vi "Subtract Coinc Stats.vi"(8 "Statistics to remove":T1, 11 "Existing statistics":i32[][](array[numeric])) -> (3 "Output":i32[][](array[numeric]))   [LabVIEW 2016]
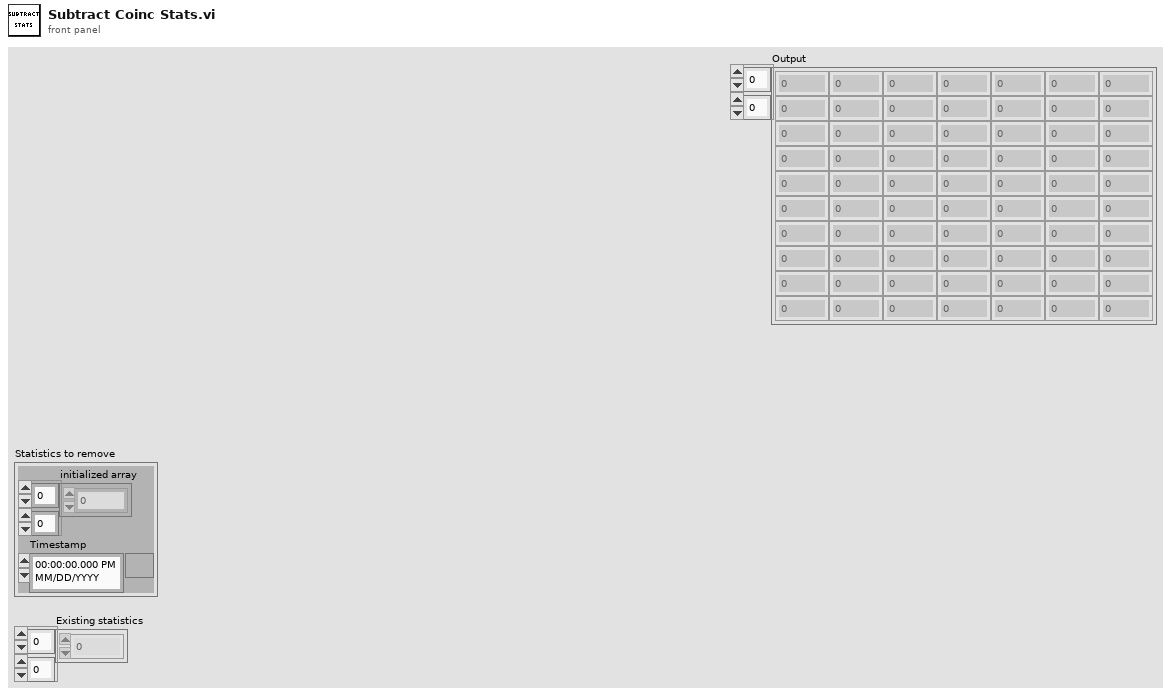
[diagram p1: front panel]
types:
  T1 = cluster{"initialized array":i16[][], "Timestamp":timestamp}
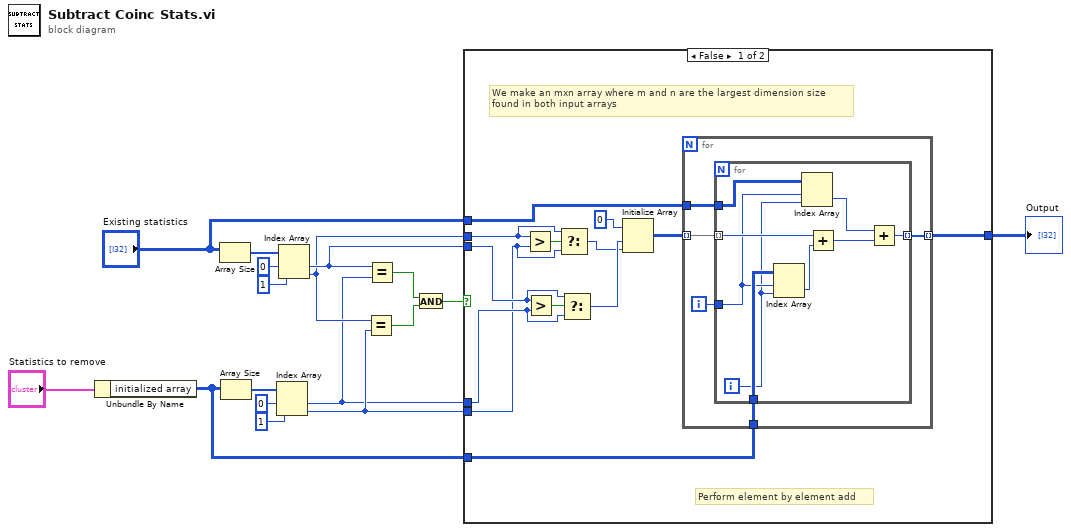
[diagram p0: block diagram]
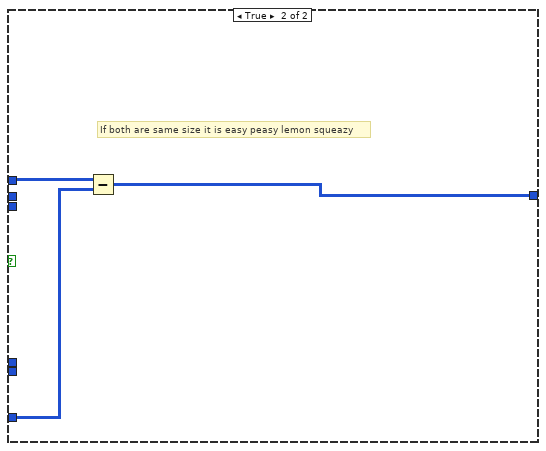
[diagram p2: hidden frame]
diagram:
  n1 = Unbundle By Name("Statistics to remove") -> ("initialized array"=w2:i16[][])
  n2 = Array Size(array="Existing statistics") -> (size(s)=w16:i32[])
  n3 = Array Size(array=w2) -> (size(s)=w11:i32[])
  n4 = Index Array(array=w11, index #1=0 ("index"), index #2=1 ("index")) -> (element #1=w4:i32, element #2=w5:i32)
  n5 = Index Array(array=w16, index #1=0 ("index"), index #2=1 ("index")) -> (element #1=w7:i32, element #2=w6:i32)
  n6 = Equal?(x=w6, y=w5) -> (x = y?=w9:bool)
  n7 = Equal?(x=w7, y=w4) -> (x = y?=w10:bool)
  n8 = And(x=w10, y=w9) -> (x .and. y?=w8:bool)
  n9 = case shown="False" w8 {
    tunnel: "Existing statistics" -> [w18 w47]
    tunnel: w2 -> [w20 w46]
    tunnel: [w19 w45] -> w1
    tunnel: w7 -> [w29 _]
    tunnel: w6 -> [w26 _]
    tunnel: w5 -> [w25 _]
    tunnel: w4 -> [w28 _]
    frame False {
      # "Perform element by element add"
      # "We make an mxn array where m and n are the largest dimension size\nfound in both input arrays"
      n10 = Greater?(x=w26, y=w25) -> (0:w27:bool)
      n11 = Greater?(x=w29, y=w28) -> (0:w30:bool)
      n12 = Select(t=w26, s=w27, f=w25) -> (s? t:f=w22:i32)
      n13 = Select(t=w29, s=w30, f=w28) -> (s? t:f=w23:i32)
      n14 = Initialize Array(0, w23, w22) -> (w21:i32[][])
      n15 = for {
        tunnel: w21 -> [w35] mode=indexing
        tunnel: w20 -> [w34]
        tunnel: [w32] -> w19 mode=indexing
        tunnel: w18 -> [w31]
        i -> [w33]
        n16 = for {
          tunnel: w35 -> [w44] mode=indexing
          tunnel: w34 -> [w43]
          tunnel: w33 -> [w39]
          tunnel: [w36] -> w32 mode=indexing
          tunnel: w31 -> [w40]
          i -> [w38]
          n17 = Index Array(array=w43, index (row)=w39, index (col)=w38) -> (element=w42:i16)
          n18 = Index Array(array=w40, index (row)=w39, index (col)=w38) -> (element=w37:i32)
          n19 = Add(x=w44, y=w42) -> (x+y=w41:i32)
          n20 = Add(x=w37, y=w41) -> (x+y=w36:i32)
        }
      }
    }
    frame True {
      # "If both are same size it is easy peasy lemon squeazy"
      n21 = Subtract(x=w47, y=w46) -> (x-y=w45:i32[][])
    }
  }
  "Output" <- w1
